vi "Parse Data Replay Loops.vi"(10 "Control Arrays":T1, 11 "Control Scalars":T5) -> (3 "DataReplay Loops":T3[](array[typedef]))   [LabVIEW 2011, in "Engine Sim System Explorer.lvlib"]
uses:
  Engine Sim System Explorer.lvlib
  <userlib>/_FPGA Interface Advanced Tools/FPGA Bitfile Utility/TypeDefs/Scalar Register Set.ctl
  <userlib>/_FPGA Interface Advanced Tools/FPGA Bitfile Utility/TypeDefs/Scalar Register.ctl
  TypeDefs/DataReplayLoopComp.ctl
  TypeDefs/DataReplayComp.ctl
  <userlib>/_FPGA Interface Advanced Tools/FPGA Bitfile Utility/TypeDefs/Array Register Set.ctl
  <userlib>/_FPGA Interface Advanced Tools/FPGA Bitfile Utility/TypeDefs/Array Register.ctl
  <vilib>/regexp/Match Regular Expression.xnode
  <userlib>/_FPGA Interface Advanced Tools/FPGA Bitfile Utility/FPGA Bitfile Utility.lvlib
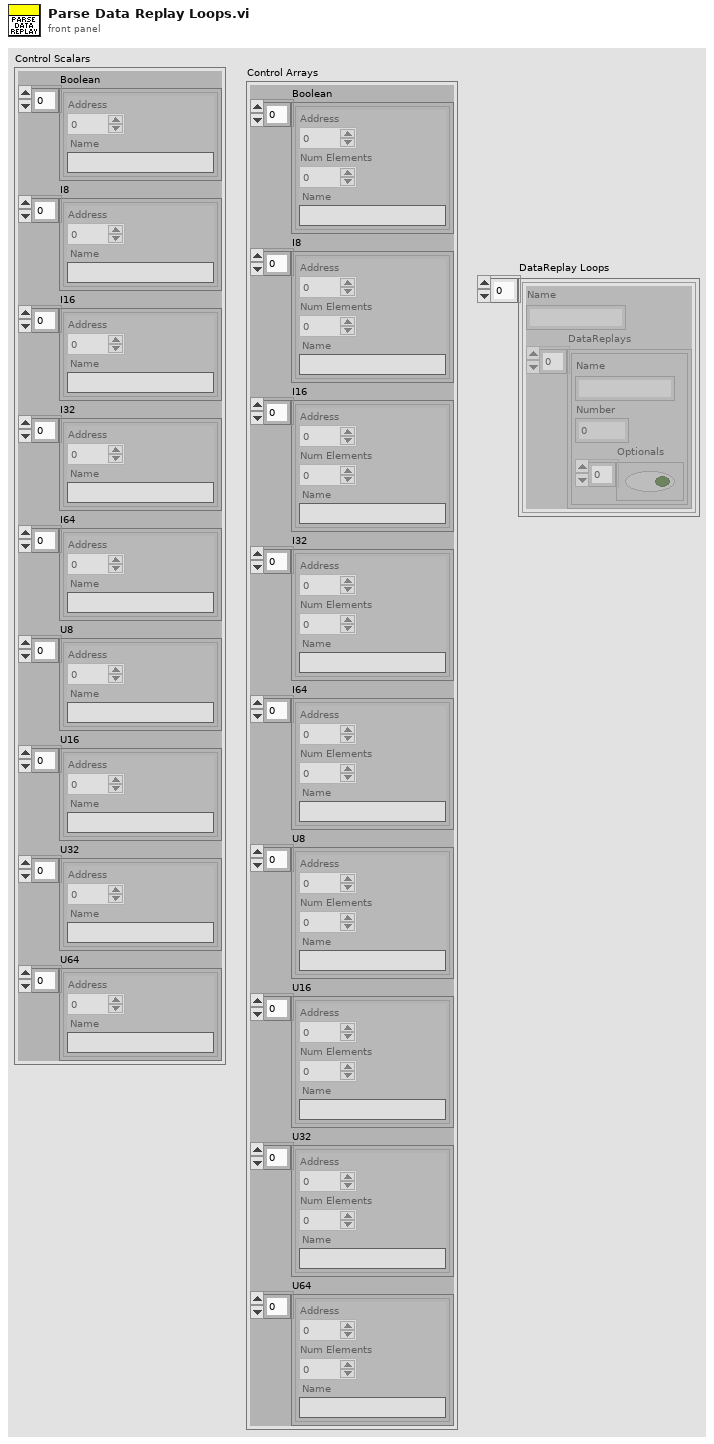
[diagram p1: front panel]
types:
  T1 = typedef "FPGA Bitfile Utility.lvlib/Array Register Set.ctl" = cluster{"Boolean":T2[], "I8":T2[], "I16":T2[], "I32":T2[], "I64":T2[], "U8":T2[], "U16":T2[], "U32":T2[], "U64":T2[]}
  T2 = typedef "FPGA Bitfile Utility.lvlib/Array Register.ctl" = cluster{"Address":u32, "Num Elements":u32, "Name":string}
  T3 = typedef "Engine Sim System Explorer.lvlib/DataReplayLoopComp.ctl" = cluster{"Name":string, "DataReplays":T4[]}
  T4 = typedef "Engine Sim System Explorer.lvlib/DataReplayComp.ctl" = cluster{"Name":string, "Number":i32, "Optionals":bool[]}
  T5 = typedef "FPGA Bitfile Utility.lvlib/Scalar Register Set.ctl" = cluster{"Boolean":T6[], "I8":T6[], "I16":T6[], "I32":T6[], "I64":T6[], "U8":T6[], "U16":T6[], "U32":T6[], "U64":T6[]}
  T6 = typedef "FPGA Bitfile Utility.lvlib/Scalar Register.ctl" = cluster{"Address":u32, "Name":string}
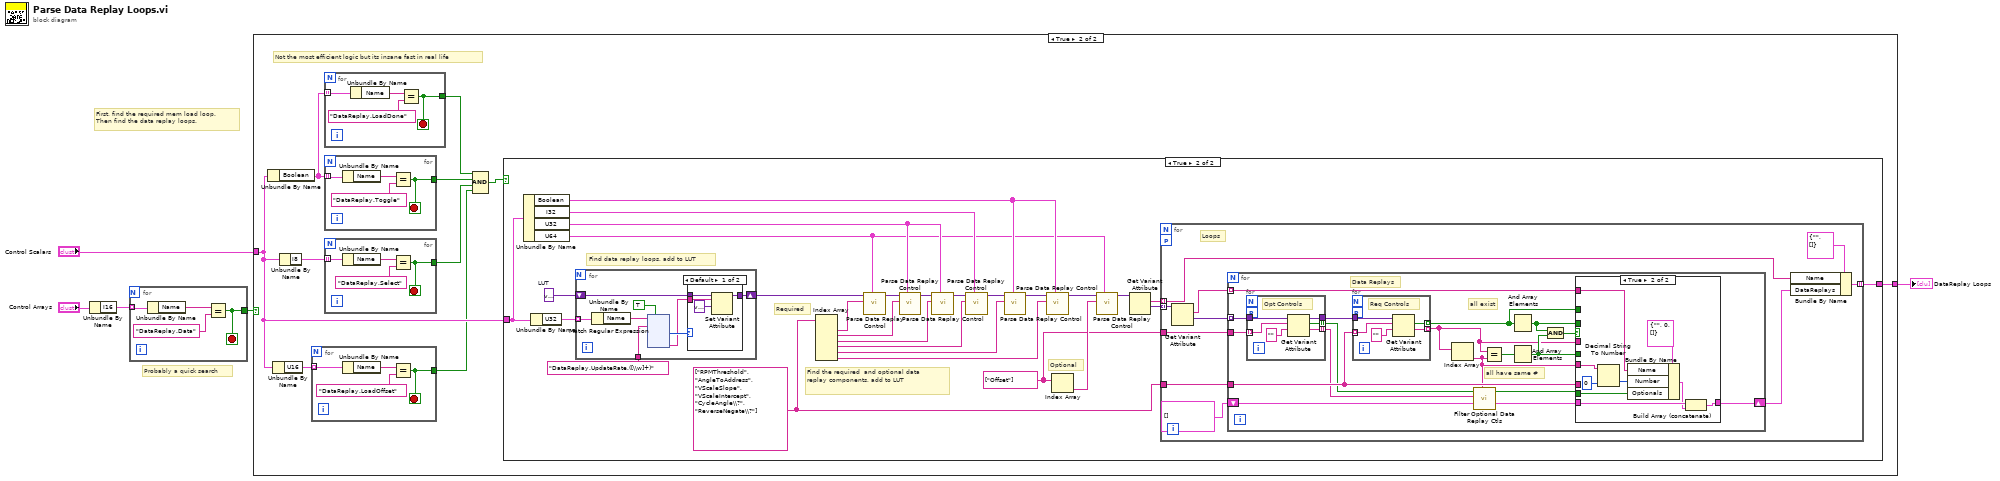
[diagram p0: block diagram]
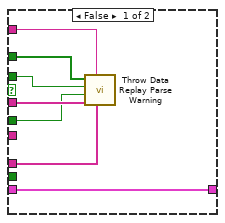
[diagram p4: hidden frame]
diagram:
  # "Probably a quick search"
  # "First, find the required mem load loop.\nThen find the data replay loops."
  n1 = Unbundle By Name("Control Arrays") -> ("I16"=w4:T2[])
  n2 = for {
    tunnel: w4 -> [w9] mode=indexing
    tunnel: [w6] -> w3
    stop <- w6 stop-if-true
    n3 = Unbundle By Name(w9) -> ("Name"=w8:string)
    n4 = Equal?(x=w8, y="DataReplay.Data") -> (x = y?=w6:bool)
  }
  n5 = case shown="True" w3 {
    tunnel: "Control Scalars" -> [_ w11]
    tunnel: [_ w13] -> w1
    frame False {
    }
    frame True {
      # "Not the most efficient logic but its insane fast in real life"
      n6 = Unbundle By Name(w11) -> ("Boolean"=w19:T6[])
      n7 = Unbundle By Name(w11) -> ("U16"=w12:T6[])
      n8 = Unbundle By Name(w11) -> ("I8"=w18:T6[])
      n9 = for {
        tunnel: w12 -> [w23] mode=indexing
        tunnel: [w20] -> w10
        stop <- w20 stop-if-true
        n10 = Unbundle By Name(w23) -> ("Name"=w22:string)
        n11 = Equal?(x=w22, y="DataReplay.LoadOffset") -> (x = y?=w20:bool)
      }
      n12 = for {
        tunnel: w19 -> [w239] mode=indexing
        tunnel: [w236] -> w17
        stop <- w236 stop-if-true
        n13 = Unbundle By Name(w239) -> ("Name"=w238:string)
        n14 = Equal?(x=w238, y="DataReplay.LoadDone") -> (x = y?=w236:bool)
      }
      n15 = for {
        tunnel: w19 -> [w243] mode=indexing
        tunnel: [w240] -> w16
        stop <- w240 stop-if-true
        n16 = Unbundle By Name(w243) -> ("Name"=w242:string)
        n17 = Equal?(x=w242, y="DataReplay.Toggle") -> (x = y?=w240:bool)
      }
      n18 = for {
        tunnel: w18 -> [w235] mode=indexing
        tunnel: [w232] -> w15
        stop <- w232 stop-if-true
        n19 = Unbundle By Name(w235) -> ("Name"=w234:string)
        n20 = Equal?(x=w234, y="DataReplay.Select") -> (x = y?=w232:bool)
      }
      n21 = Compound Arithmetic op=AND(w17, w16, w15, w10) -> (w14:bool)
      n22 = case shown="True" w14 {
        tunnel: w11 -> [_ w48]
        tunnel: [_ w42] -> w13
        frame False {
        }
        frame True {
          w24 = string[] ["Offset"]
          w38 = string[] ["RPMThreshold", "AngleToAddress", "VScaleSlope", "VScaleIntercept", "CycleAngle\\?", "ReverseNegate\\?"]
          w50 = variant  # LUT
          # "Optional"
          # "Required"
          # "Find the required  and optional data replay components, add to LUT"
          # "Find data replay loops, add to LUT"
          n23 = Unbundle By Name(w48) -> ("Boolean"=w29:T6[], "I32"=w34:T6[], "U32"=w36:T6[], "U64"=w26:T6[])
          n24 = Unbundle By Name(w48) -> ("U32"=w51:T6[])
          n25 = for {
            tunnel: w51 -> [w113] mode=indexing
            shift-right: [w109] -> w47
            shift-left: w50 -> [w110]
            tunnel: "DataReplay.UpdateRate.([\\w]+)" ("regular expression") -> [w107]
            n26 = Unbundle By Name(w113) -> ("Name"=w112:string)
            n27 = xnode "Match Regular Expression"("input string"=w112, "regular expression"=w107, "ignore case? (F)"=TRUE) -> ("offset past match"=w111:i32, "submatch 1"=w106:string)  [unwired: 3 in, 4 out]
            n28 = case shown="Default" w111 {
              tunnel: w110 -> [w117 w118]
              tunnel: w106 -> [w116 _]
              tunnel: [w115 w118] -> w109
              frame Default {
                n29 = Set Variant Attribute(Variant=w117, name=w116, value=variant ("LUT")) -> (Variant out=w115:variant)  [unwired: 1 in, 2 out]
              }
              frame -1 {
              }
            }
          }
          n30 = Index Array(array=w38) -> (element #1=w41:string, element #2=w40:string, element #3=w39:string, element #4=w35:string, element #5=w32:string, element #6=w28:string)  [unwired: 6 in]
          n31 = call "Parse Data Replay Control.vi"("Controls"=w26, "Control Name"=w41, "LUT in"=w47) -> ("LUT out"=w46:variant)  [unwired: 8 in]
          n32 = call "Parse Data Replay Control.vi"("Controls"=w36, "Control Name"=w40, "LUT in"=w46) -> ("LUT out"=w45:variant)  [unwired: 8 in]
          n33 = call "Parse Data Replay Control.vi"("Controls"=w36, "Control Name"=w39, "LUT in"=w45) -> ("LUT out"=w37:variant)  [unwired: 8 in]
          n34 = call "Parse Data Replay Control.vi"("Controls"=w34, "Control Name"=w35, "LUT in"=w37) -> ("LUT out"=w33:variant)  [unwired: 8 in]
          n35 = call "Parse Data Replay Control.vi"("Controls"=w29, "Control Name"=w32, "LUT in"=w33) -> ("LUT out"=w31:variant)  [unwired: 8 in]
          n36 = call "Parse Data Replay Control.vi"("Controls"=w29, "Control Name"=w28, "LUT in"=w31) -> ("LUT out"=w30:variant)  [unwired: 8 in]
          n37 = Index Array(array=w24) -> (element=w25:string)  [unwired: 1 in]
          n38 = call "Parse Data Replay Control.vi"("Controls"=w26, "Control Name"=w25, "LUT in"=w30) -> ("LUT out"=w27:variant)  [unwired: 8 in]
          n39 = Get Variant Attribute(Variant=w27) -> (names=w44:string[], values=w43:variant[])  [unwired: 3 in, 2 out]
          n40 = for {
            tunnel: w44 -> [w57] mode=indexing
            tunnel: w43 -> [w61] mode=indexing
            tunnel: w38 -> [w56]
            tunnel: [w53] -> w42 mode=indexing
            tunnel: w24 -> [w52]
            workers-P: _ -> [_]
            # "Loops"
            n41 = Get Variant Attribute(Variant=w61) -> (names=w60:string[], values=w59:variant[])  [unwired: 3 in, 2 out]
            n42 = for {
              tunnel: w60 -> [w74] mode=indexing
              tunnel: w59 -> [w69] mode=indexing
              tunnel: w56 -> [w72]
              shift-right: [w75] -> w54
              shift-left: T4[] [] -> [w76]
              tunnel: w52 -> [w67]
              # "all have same #"
              # "all exist"
              # "Data Replays"
              n43 = for {
                tunnel: w67 -> [w83] mode=indexing
                tunnel: [w82] -> w65 mode=indexing
                tunnel: [w80] -> w64 mode=indexing
                tunnel: w69 -> [w84]
                tunnel: [w79] -> w68
                workers-P: _ -> [_]
                # "Opt Controls"
                n44 = Get Variant Attribute(Variant=w84, name=w83, default value (empty Variant)="") -> (duplicate Variant=w79:variant, found=w82:bool, value=w80:string)  [unwired: 1 in, 1 out]
              }
              n45 = for {
                tunnel: w68 -> [w105]
                tunnel: w72 -> [w104] mode=indexing
                tunnel: [w103] -> w73 mode=indexing
                tunnel: [w101] -> w66 mode=indexing
                workers-P: _ -> [_]
                # "Req Controls"
                n46 = Get Variant Attribute(Variant=w105, name=w104, default value (empty Variant)="") -> (found=w103:bool, value=w101:string)  [unwired: 1 in, 2 out]
              }
              n47 = Index Array(array=w66) -> (element=w63:string)  [unwired: 1 in]
              n48 = call "Filter Optional Data Replay Ctls.vi"("Replay#"=w63, "Numbers"=w64, "Found in"=w65) -> ("Found out"=w62:bool[])  [unwired: 8 in]
              n49 = Equal?(x=w66, y=w63) -> (x = y?=w78:bool[])
              n50 = And Array Elements(Boolean array=w73) -> (logical AND=w71:bool)
              n51 = And Array Elements(Boolean array=w78) -> (logical AND=w70:bool)
              n52 = And(x=w71, y=w70) -> (x .and. y?=w77:bool)
              n53 = case shown="True" w77 {
                tunnel: w76 -> [w91 w100]
                tunnel: [w91 w98] -> w75
                tunnel: w74 -> [w87 w97]
                tunnel: w63 -> [_ w94]
                tunnel: w73 -> [w88 _]
                tunnel: w66 -> [w90 _]
                tunnel: w72 -> [w86 _]
                tunnel: w71 -> [w89 _]
                tunnel: w70 -> [w85 _]
                tunnel: w62 -> [_ w92]
                frame False {
                  n54 = call "Throw Data Replay Parse Warning.vi"("Controls"=w86, "Replay"=w87, "Found Numbers"=w90, "All numbers same?"=w85, "All controls present?"=w89, "Found Controls"=w88) -> ()  [unwired: 6 in]
                }
                frame True {
                  n55 = Decimal String To Number(string=w94, default (0L)=0 ("default (0 I32)")) -> (number=w95:i32)  [unwired: 1 in, 1 out]
                  n56 = Bundle By Name(cluster=T4 {"Name"="", "Number"=0, "Optionals"=[]} ("DataReplay"), "Name"=w97, "Number"=w95, "Optionals"=w92) -> (w96:T4)
                  n57 = Build Array (concatenate)(w100, w96) -> (w98:T4[])
                }
              }
            }
            n58 = Bundle By Name(cluster=T3 {"Name"="", "DataReplays"=[]} ("DataReplayLoop"), "Name"=w57, "DataReplays"=w54) -> (w53:T3)
          }
        }
      }
    }
  }
  "DataReplay Loops" <- w1
